vi "Insert Into Array.vi"() -> ()   [LabVIEW 2012]
panel:
  out "Output 2D Array":i32[][](array[numeric])
  out "Output 1D Array":i32[](array[numeric])
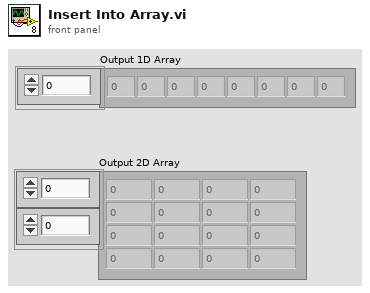
[diagram p1: front panel]
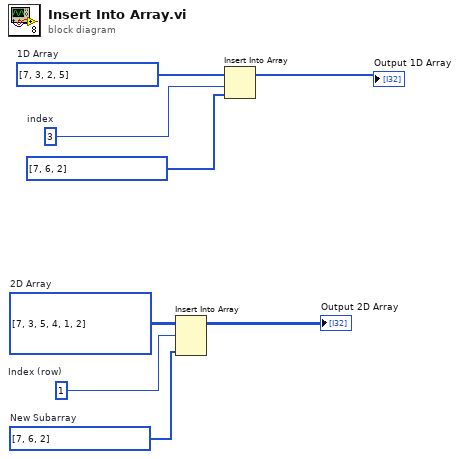
[diagram p0: block diagram]
diagram:
  w2 = i32[] [7, 6, 2]  # New Subarray
  w4 = 1  # Index (row)
  w7 = 3  # index
  w5 = i32[][] [[7, 3, 5], [4, 1, 2]]  # 2D Array
  w8 = i32[] [7, 3, 2, 5]  # 1D Array
  n1 = Insert Into Array "Insert Into Array"(array=w5, index (row)=w4, new element=w2) -> (→"Output 2D Array":i32[][])  [unwired: 1 in]
  n2 = Insert Into Array "Insert Into Array"(array=w8, index=w7, new element=i32[] [7, 6, 2]) -> (→"Output 1D Array":i32[])
